vi "Delete Process and Close SV.vi"(8 "error in (no error)":errorcluster, 10 "Array":refnum<k21>[](array[refnum]), 11 "process name":string) -> (0 "error out":errorcluster)   [LabVIEW 2021, in "Dynamic Shared Variables.lvlib"]
uses:
  Dynamic Shared Variables.lvlib
  <vilib>/lvdsc/NI_DSC.lvlib
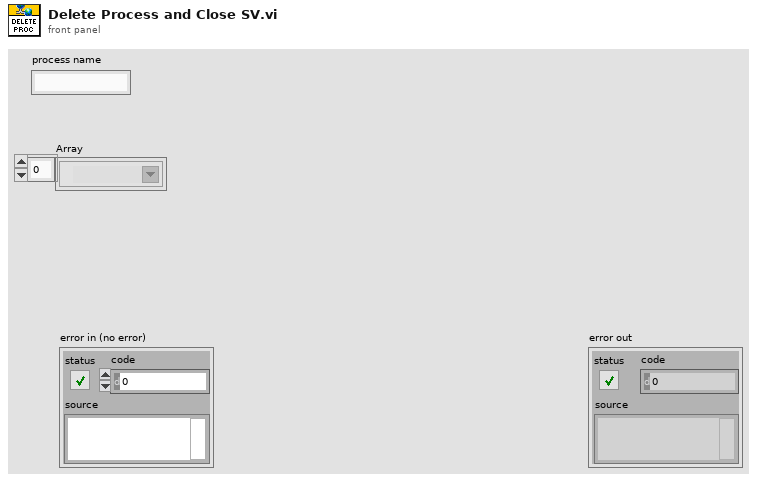
[diagram p1: front panel]
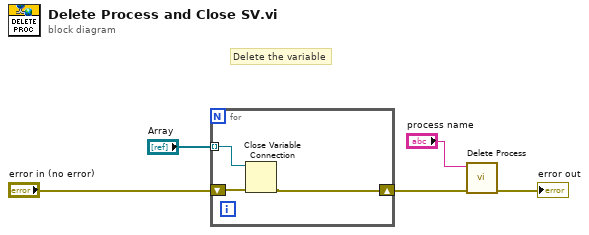
[diagram p0: block diagram]
diagram:
  # "Delete the variable"
  n1 = for {
    tunnel: "Array" -> [w8] mode=indexing
    shift-right: [w6] -> w4
    shift-left: "error in (no error)" -> [w7]
    n2 = Close Variable Connection(8:w7, 11:w8) -> (0:w6:errorcluster)
  }
  n3 = call <vilib>:"Delete Process.vi"("error in (no error)"=w4, "process name"="process name") -> ("error out"=→"error out":errorcluster)  [unwired: 9 in]
